vi "Test 5.vi"() -> ()   [LabVIEW 2024, in "Test Class 1.lvclass"]
uses:
  Test Class 1.lvclass
panel:
  in  "Numeric":dbl
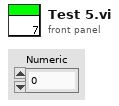
[diagram p1: front panel]
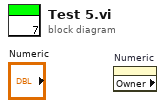
[diagram p0: block diagram]
diagram:
  n1 = property on="Numeric" class="DigNum (strict)" props=["Owner"]() -> ()  [unwired: 2 in, 3 out]
